vi "Calibrate.vi"(8 "error in (no error)":errorcluster, 11 "BME_DG_System in":refnum<class "BME_DG_System.lvclass">) -> (0 "error out":errorcluster, 3 "BME_DG_System out":refnum<class "BME_DG_System.lvclass">)   [LabVIEW 2009, in "POLARIS BME DG.lvlib" / "BME_DG_System.lvclass"]
uses:
  BME_DG_System.lvclass
  BME_DG_System.lvclass/BME_DG_System.ctl
  LV-BME Interface/BME_DG_MasterOrSlave.ctl
  BME_DG_Base/BME_DG_Base.lvclass
  POLARIS BME DG.lvlib
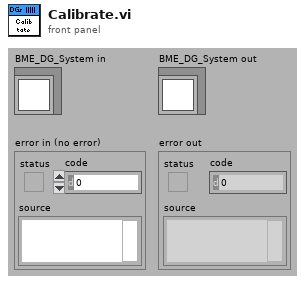
[diagram p1: front panel]
types:
  T1 = typedef "POLARIS BME DG.lvlib/BME_DG_MasterOrSlave.ctl" = enum16{"Unknown", "Master", "Slave"}
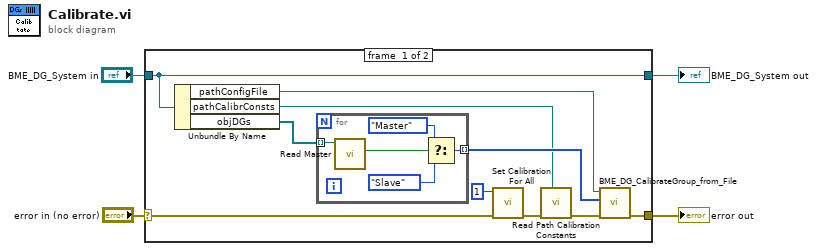
[diagram p0: block diagram]
diagram:
  n1 = case shown="No Error" "error in (no error)" {
    selector: "error in (no error)" -> [w9 w21]
    tunnel: [w13 w21] -> w3
    tunnel: [w14 w20] -> w1
    tunnel: "BME_DG_System in" -> [w14 w20]
    frame #0 {
      n2 = Unbundle By Name(w14) -> ("pathConfigFile"=w6:path, "pathCalibrConsts"=w5:path, "objDGs"=w12:refnum<class "BME_DG_Base.lvclass">[])
      n3 = for {
        tunnel: w12 -> [w19] mode=indexing
        tunnel: [w15] -> w11 mode=indexing
        n4 = call-dynamic "Read Master.vi"("BME_DG_Base in"=w19) -> ("Master?"=w18:bool)  [unwired: 7 in, 3 out]
        n5 = Select(t=BME_DG_MasterOrSlave."Master" ("BME_DG_MasterOrSlave"), s=w18, f=BME_DG_MasterOrSlave."Slave" ("BME_DG_MasterOrSlave")) -> (s? t:f=w15:T1)
      }
      n6 = call "Set Calibration For All.vi"("error in (no error)"=w9, "Calibration Level"=u32 1) -> ("error out"=w8:errorcluster)  [unwired: 9 in]
      n7 = call "Read Path Calibration Constants.vi"("Path"=w5, "error in (no error)"=w8) -> ("error out"=w7:errorcluster)  [unwired: 9 in]
      n8 = call "BME_DG_CalibrateGroup_from_File.vi"("error in (no error)"=w7, "p_MasterOrSlave"=w11, "Path"=w6) -> ("error out"=w13:errorcluster)  [unwired: 7 in, 1 out]
    }
    frame #1 {
    }
  }
  "error out" <- w3
  "BME_DG_System out" <- w1
